vi "CRYGet Two Units Rows.vi"(6 "Phase":bool[](array[boolean]), 8 "pGraph VI In":refnum<vi>, 9 "New Rows In":i32[](array[numeric]), 10 "Old Rows In":i32[](array[numeric]), 11 "Type":enum16{"Curves", "Values", "Results", "WFM"}(ring)) -> (0 "Unit2":string, 1 "Unit1":string, 3 "All Rows Out":i32[](array[numeric]), 4 "Two Units":i32, 5 "New Rows Out":i32[](array[numeric]), 7 "New Exist?":bool)   [LabVIEW 2013]
panel:
  out "Find1":bool
  out "Message":bool
  out "Find2":bool
  out "Unit Flag":i32[](array[numeric])
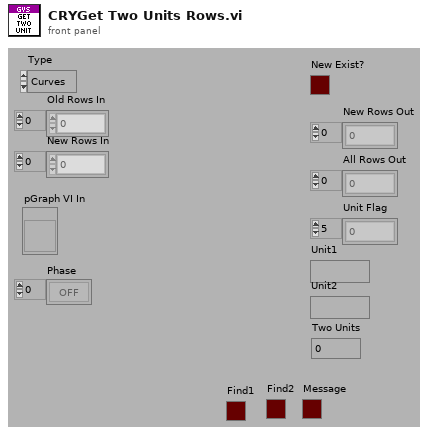
[diagram p1: front panel]
types:
  T1 = enum16{"OK", "Yes", "YesNo", "YesNoCancel", "ReplaceAppend"}
  T2 = typedef "CRYData Cluster.ctl" = cluster{"Name":string, "Curve":cluster{"x":dbl, "y":dbl, "z":dbl}[], "X data":u16, "Y data":u16, "Z data":u16, "X axis":u16, "Y axis":u16, "Z axis":u16, "X unit":string, "Y unit":string, "Z unit":string, "X dB ref":dbl, "Y dB ref":dbl, "Z dB ref":dbl, "single val":bool, "protected":bool, "display X":bool, "display Y":bool, "display Z":bool, "Test Info":string, "Step No.":i32, "Plot Settings":cluster{"Color":u32, "Interpolation":u8, "Point Style":u8, "Line Style":u8, "Point Color":u32, "Line Width":u8, "Bar Plot Style":u8, "Fill To":i16}, "AutoProtect":bool}
  T3 = typedef "CRYWaveform Cluster.ctl" = cluster{"Waveform":cluster{"X0":dbl, "dX":dbl, "Y":sgl[]}, "X data":u16, "Y data":u16, "Y axis":u16, "X unit":string, "Y unit":string, "Y dB ref":dbl, "display Y":bool, "display X":bool, "Overload?":bool, "Test Info":string, "Step No.":i32, "Name":string, "protected":bool, "Sqc history":string[], "Signal Channel ID":i32, "Plot Settings":cluster{"Color":u32, "Interpolation":u8, "Point Style":u8, "Line Style":u8, "Point Color":u32, "Line Width":u8, "Bar Plot Style":u8, "Fill To":i16}, "AutoProtect":bool}
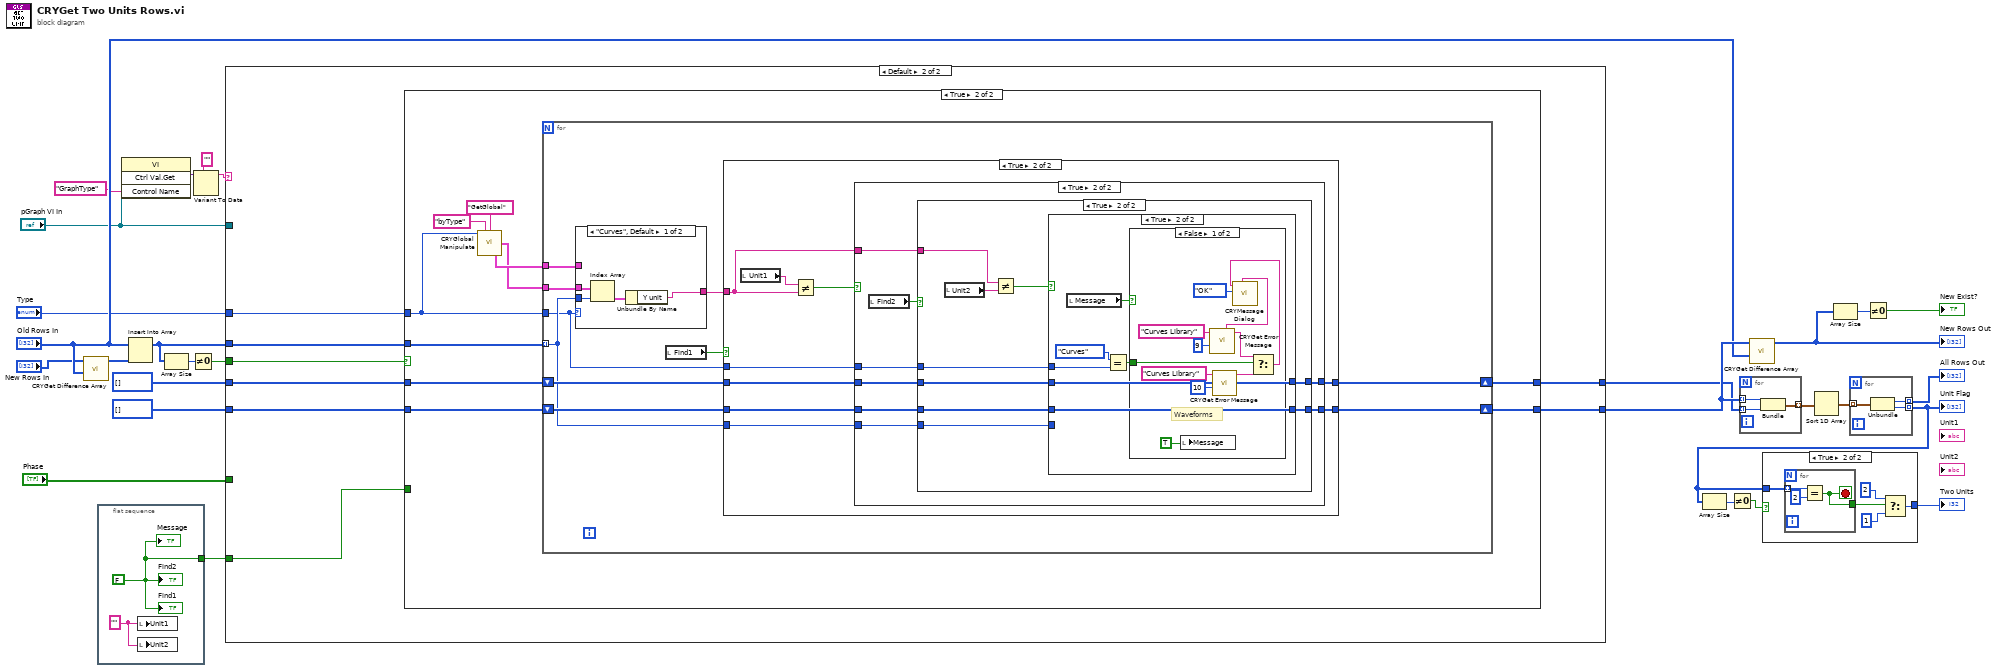
[diagram p0: block diagram]
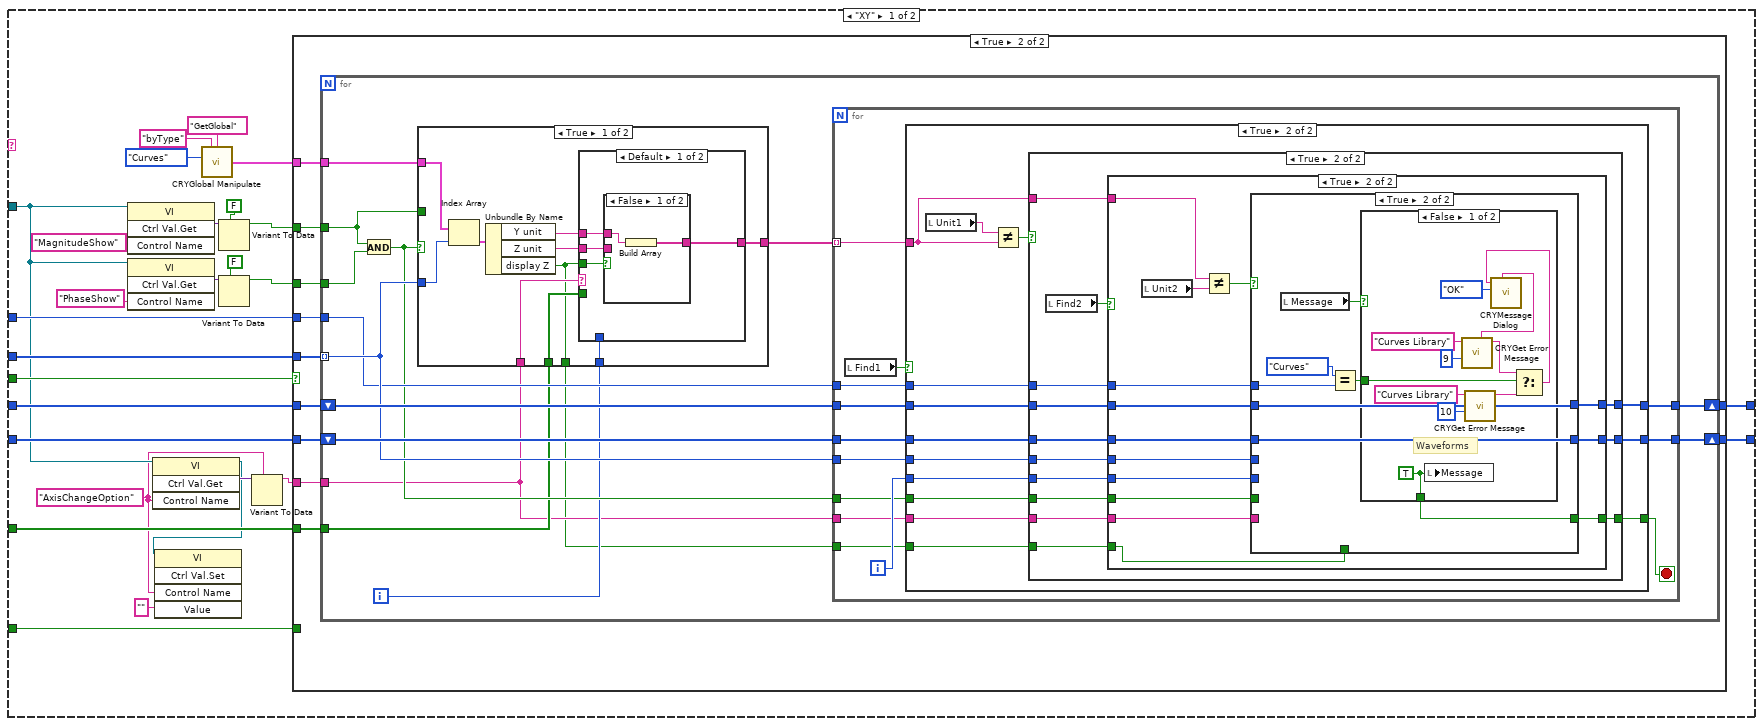
[diagram p2: hidden frame]
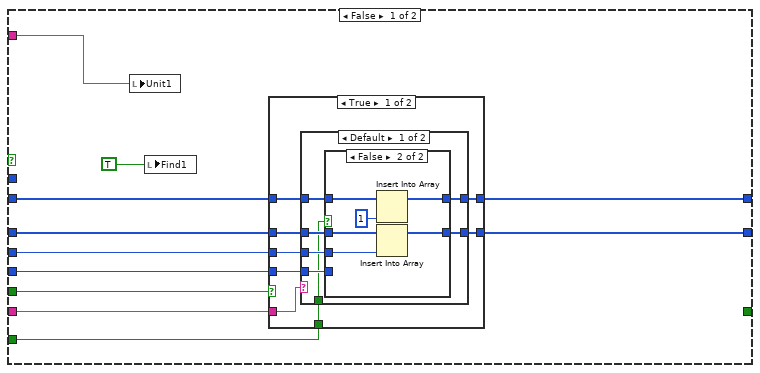
[diagram p4: hidden frame]
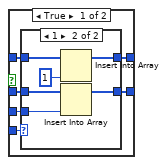
[diagram p5: hidden frame]
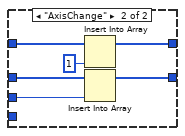
[diagram p7: hidden frame]
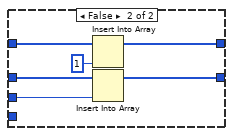
[diagram p8: hidden frame]
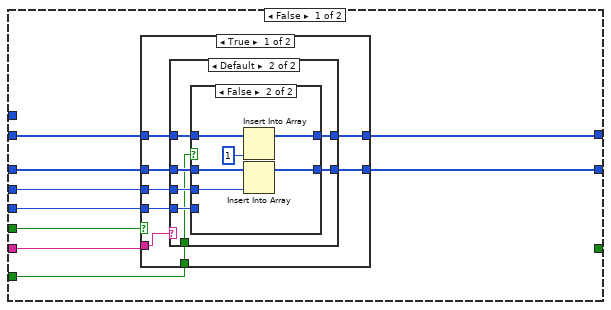
[diagram p9: hidden frame]
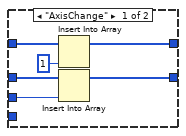
[diagram p10: hidden frame]
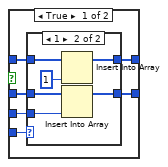
[diagram p11: hidden frame]
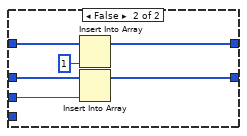
[diagram p13: hidden frame]
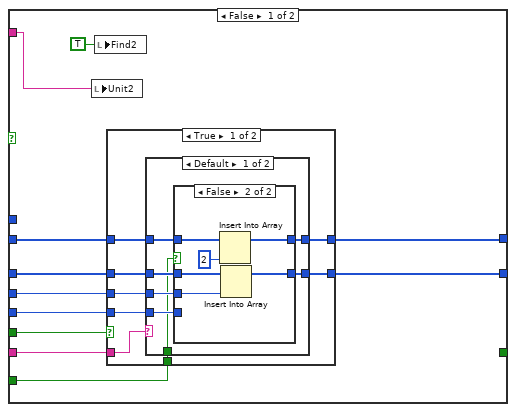
[diagram p14: hidden frame]
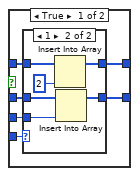
[diagram p15: hidden frame]
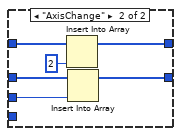
[diagram p17: hidden frame]
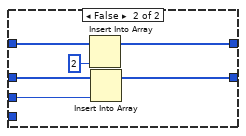
[diagram p18: hidden frame]
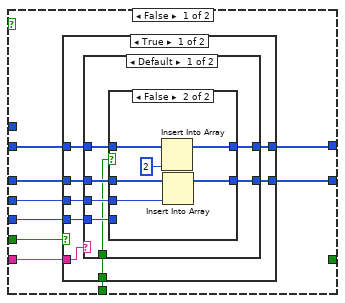
[diagram p19: hidden frame]
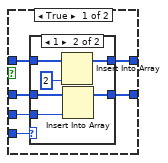
[diagram p20: hidden frame]
diagram:
  n1 = call "CRYGet Difference Array.vi"("Array 2"="Old Rows In", "Array 1"="New Rows In") -> ("Diff Out"=w16:i32[])  [unwired: 3 in, 6 out]
  n2 = flat-sequence {
    tunnel: [w30] -> w28
    frame #0 {
      w29 = "" ("Unit Y1")
      w30 = FALSE ("Find")
      n3 = local write "Unit1"(w29) -> ()
      n4 = local write "Unit2"(w29) -> ()
      "Find2" <- w30
      "Message" <- w30
      "Find1" <- w30
    }
  }
  n5 = invoke class="VI" method="Ctrl Val.Get"(reference="pGraph VI In", "Control Name"="GraphType") -> ("Get Control Value Variant"=w6:variant)  [unwired: 2 in, 3 out]
  n6 = Insert Into Array(array="Old Rows In", new element=w16) -> (w9:i32[])  [unwired: 1 in]
  n7 = Array Size(array=w9) -> (size(s)=w10:i32)
  n8 = Not Equal To 0?(x=w10) -> (x != 0?=w8:bool)
  n9 = Variant To Data(type="" ("Control Name"), Variant=w6) -> (data=w3:string)  [unwired: 1 in, 1 out]
  n10 = case shown="Default" w3 {
    tunnel: w28 -> [w57 w432]
    tunnel: i32[] [] ("Selected Row In") -> [w56 w431]
    tunnel: i32[] [] ("Selected Row In") -> [w55 w430]
    tunnel: [w54 w429] -> w23
    tunnel: [w53 w428] -> w22
    tunnel: w9 -> [w52 w427]
    tunnel: w8 -> [w51 w426]
    tunnel: "Type" -> [w50 w425]
    tunnel: "pGraph VI In" -> [w40 _]
    tunnel: "Phase" -> [w38 _]
    frame "XY" {
      w35 = "AxisChangeOption" ("Control Name")
      n11 = invoke class="VI" method="Ctrl Val.Get"(reference=w40, "Control Name"="MagnitudeShow") -> ("Get Control Value Variant"=w45:variant)  [unwired: 2 in, 3 out]
      n12 = invoke class="VI" method="Ctrl Val.Get"(reference=w40, "Control Name"="PhaseShow") -> ("Get Control Value Variant"=w46:variant)  [unwired: 2 in, 3 out]
      n13 = invoke class="VI" method="Ctrl Val.Get"(reference=w40, "Control Name"=w35) -> (reference out=w37:refnum<vi>, "Get Control Value Variant"=w41:variant)  [unwired: 2 in, 2 out]
      n14 = invoke class="VI" method="Ctrl Val.Set"(reference=w37, "Control Name"=w35, "Value"="" ("Control Name")) -> ()  [unwired: 2 in, 5 out]
      n15 = call "CRYGlobal Manipulate.vi"("Type"=enum16{"Curves", "Values", "Results", "WFM"}."Curves", "sOption"="byType", "sAction"="GetGlobal") -> ("Curves Out"=w31:T2[])  [unwired: 6 in, 6 out]
      n16 = Variant To Data(type=FALSE ("Find"), Variant=w45) -> (data=w43:bool)  [unwired: 1 in, 1 out]
      n17 = Variant To Data(type=FALSE ("Find"), Variant=w46) -> (data=w42:bool)  [unwired: 1 in, 1 out]
      n18 = Variant To Data(type=w35, Variant=w41) -> (data=w39:string)  [unwired: 1 in, 1 out]
      n19 = case shown="True" w51 {
        tunnel: w57 -> [_ _]
        tunnel: w56 -> [w58 w70]
        tunnel: w55 -> [w59 w69]
        tunnel: [w59 w68] -> w54
        tunnel: [w58 w67] -> w53
        tunnel: w52 -> [_ w66]
        tunnel: w50 -> [_ w65]
        tunnel: w43 -> [_ w63]
        tunnel: w42 -> [_ w62]
        tunnel: w31 -> [_ w64]
        tunnel: w39 -> [_ w61]
        tunnel: w38 -> [_ w60]
        frame False {
        }
        frame True {
          n20 = for {
            tunnel: w66 -> [w81] mode=indexing
            shift-right: [w84] -> w67
            shift-left: w70 -> [w85]
            shift-right: [w82] -> w68
            shift-left: w69 -> [w83]
            tunnel: w65 -> [w80]
            tunnel: w64 -> [w75]
            tunnel: w63 -> [w79]
            tunnel: w62 -> [w78]
            tunnel: w61 -> [w73]
            tunnel: w60 -> [w76]
            i -> [w74]
            n21 = And(x=w79, y=w78) -> (x .and. y?=w77:bool)
            n22 = case shown="True" w77 {
              tunnel: w81 -> [w396 w424]
              tunnel: [w395 w418] -> w72
              tunnel: w79 -> [_ w419]
              tunnel: w73 -> [w391 _]
              tunnel: w76 -> [w390 _]
              tunnel: w75 -> [w389 w417]
              tunnel: w74 -> [w388 _]
              tunnel: [w387 FALSE ("display Z")] -> w71
              frame True {
                n23 = Index Array(array=w389, index=w396) -> (element=w394:T2)
                n24 = Unbundle By Name(w394) -> ("Y unit"=w393:string, "Z unit"=w392:string, "display Z"=w387:bool)
                n25 = case shown="Default" w391 {
                  tunnel: [w400 w411] -> w395
                  tunnel: w393 -> [w399 w410]
                  tunnel: w392 -> [w398 w409]
                  tunnel: w387 -> [w397 _]
                  tunnel: w390 -> [_ w408]
                  tunnel: w388 -> [_ w406]
                  frame Default {
                    n26 = case shown="False" w397 {
                      tunnel: [w401 w403] -> w400
                      tunnel: w399 -> [w402 w404]
                      tunnel: w398 -> [_ w405]
                      frame False {
                        n27 = Build Array(w402) -> (w401:string[])
                      }
                      frame True {
                        n28 = Build Array(w404, w405) -> (w403:string[])
                      }
                    }
                  }
                  frame "AxisChange" {
                    n29 = Index Array(array=w408, index=w406) -> (element=w407:bool)
                    n30 = case shown="True" w407 {
                      tunnel: [w413 w414] -> w411
                      tunnel: w410 -> [_ w415]
                      tunnel: w409 -> [w412 _]
                      frame False {
                        n31 = Build Array(w412) -> (w413:string[])
                      }
                      frame True {
                        n32 = Build Array(w415) -> (w414:string[])
                      }
                    }
                  }
                }
              }
              frame False {
                n33 = Index Array(array=w417, index=w424) -> (element=w422:T2)
                n34 = Unbundle By Name(w422) -> ("Y unit"=w421:string, "Z unit"=w420:string)
                n35 = Select(t=w421, s=w419, f=w420) -> (s? t:f=w423:string)
                n36 = Build Array(w423) -> (w418:string[])
              }
            }
            n37 = for {
              tunnel: w85 -> [w98]
              tunnel: [w97] -> w84
              tunnel: w83 -> [w96]
              tunnel: [w95] -> w82
              tunnel: w81 -> [w94]
              tunnel: w72 -> [w93] mode=indexing
              tunnel: w80 -> [w91]
              tunnel: w77 -> [w89]
              tunnel: w73 -> [w88]
              tunnel: w71 -> [w86]
              i -> [w90]
              stop <- w87 stop-if-true
              n38 = local read "Find1"() -> (w92:bool)
              n39 = case shown="True" w92 {
                tunnel: w93 -> [w104 w170]
                tunnel: [w108 w167] -> w97
                tunnel: w98 -> [w109 w168]
                tunnel: w96 -> [w107 w166]
                tunnel: [w106 w165] -> w95
                tunnel: w94 -> [w105 w164]
                tunnel: w91 -> [_ w163]
                tunnel: w90 -> [w102 w161]
                tunnel: w89 -> [w101 w160]
                tunnel: w88 -> [w100 w159]
                tunnel: [_ w158] -> w87
                tunnel: w86 -> [w99 w157]
                frame False {
                  n40 = local write "Unit1"(w104) -> ()
                  n41 = local write "Find1"(TRUE) -> ()
                  n42 = case shown="True" w101 {
                    tunnel: w109 -> [w117 w156]
                    tunnel: [w116 w155] -> w108
                    tunnel: w107 -> [w115 w154]
                    tunnel: [w114 w153] -> w106
                    tunnel: w105 -> [w113 w152]
                    tunnel: w102 -> [w112 _]
                    tunnel: w100 -> [w111 _]
                    tunnel: w99 -> [w110 _]
                    frame True {
                      n43 = case shown="Default" w111 {
                        tunnel: w117 -> [w124 w150]
                        tunnel: [w123 w149] -> w116
                        tunnel: w115 -> [w122 w148]
                        tunnel: [w121 w147] -> w114
                        tunnel: w113 -> [w120 w146]
                        tunnel: w112 -> [w119 _]
                        tunnel: w110 -> [w118 _]
                        frame Default {
                          n44 = case shown="False" w118 {
                            tunnel: w124 -> [w130 w144]
                            tunnel: [w129 w143] -> w123
                            tunnel: w122 -> [w128 w142]
                            tunnel: [w127 w141] -> w121
                            tunnel: w120 -> [w126 w140]
                            tunnel: w119 -> [w125 _]
                            frame True {
                              n45 = case shown="1" w125 {
                                tunnel: w130 -> [w132 w138]
                                tunnel: [w132 w137] -> w129
                                tunnel: w128 -> [w131 w136]
                                tunnel: [w131 w135] -> w127
                                tunnel: w126 -> [_ w134]
                                frame 0, Default {
                                }
                                frame 1 {
                                n46 = Insert Into Array(array=w138, new element=1 ("new element/subarray")) -> (w137:i32[])  [unwired: 1 in]
                                n47 = Insert Into Array(array=w136, new element=w134) -> (w135:i32[])  [unwired: 1 in]
                                }
                              }
                            }
                            frame False {
                              n48 = Insert Into Array(array=w144, new element=1 ("new element/subarray")) -> (w143:i32[])  [unwired: 1 in]
                              n49 = Insert Into Array(array=w142, new element=w140) -> (w141:i32[])  [unwired: 1 in]
                            }
                          }
                        }
                        frame "AxisChange" {
                          n50 = Insert Into Array(array=w150, new element=1 ("new element/subarray")) -> (w149:i32[])  [unwired: 1 in]
                          n51 = Insert Into Array(array=w148, new element=w146) -> (w147:i32[])  [unwired: 1 in]
                        }
                      }
                    }
                    frame False {
                      n52 = Insert Into Array(array=w156, new element=1 ("new element/subarray")) -> (w155:i32[])  [unwired: 1 in]
                      n53 = Insert Into Array(array=w154, new element=w152) -> (w153:i32[])  [unwired: 1 in]
                    }
                  }
                }
                frame True {
                  n54 = local read "Unit1"() -> (w169:string)
                  n55 = Not Equal?(x=w169, y=w170) -> (x != y?=w162:bool)
                  n56 = case shown="True" w162 {
                    tunnel: w170 -> [_ w239]
                    tunnel: w168 -> [w179 w236]
                    tunnel: [w178 w238] -> w167
                    tunnel: w166 -> [w177 w235]
                    tunnel: [w176 w234] -> w165
                    tunnel: w164 -> [w175 w233]
                    tunnel: w163 -> [_ w232]
                    tunnel: w161 -> [w174 w231]
                    tunnel: w160 -> [w173 w230]
                    tunnel: w159 -> [w172 w229]
                    tunnel: [_ w228] -> w158
                    tunnel: w157 -> [w171 w227]
                    frame False {
                      n57 = case shown="True" w173 {
                        tunnel: w179 -> [w187 w226]
                        tunnel: [w186 w225] -> w178
                        tunnel: w177 -> [w185 w224]
                        tunnel: [w184 w223] -> w176
                        tunnel: w175 -> [w183 w222]
                        tunnel: w174 -> [w182 _]
                        tunnel: w172 -> [w181 _]
                        tunnel: w171 -> [w180 _]
                        frame True {
                          n58 = case shown="Default" w181 {
                            tunnel: w187 -> [w193 w200]
                            tunnel: [w192 w199] -> w186
                            tunnel: w185 -> [w191 w198]
                            tunnel: [w190 w197] -> w184
                            tunnel: w183 -> [w189 w196]
                            tunnel: w182 -> [_ w195]
                            tunnel: w180 -> [_ w194]
                            frame "AxisChange" {
                              n59 = Insert Into Array(array=w193, new element=1 ("new element/subarray")) -> (w192:i32[])  [unwired: 1 in]
                              n60 = Insert Into Array(array=w191, new element=w189) -> (w190:i32[])  [unwired: 1 in]
                            }
                            frame Default {
                              n61 = case shown="False" w194 {
                                tunnel: w200 -> [w206 w220]
                                tunnel: [w205 w219] -> w199
                                tunnel: w198 -> [w204 w218]
                                tunnel: [w203 w217] -> w197
                                tunnel: w196 -> [w202 w216]
                                tunnel: w195 -> [w201 _]
                                frame True {
                                n62 = case shown="1" w201 {
                                tunnel: w206 -> [w208 w213]
                                tunnel: [w208 w212] -> w205
                                tunnel: w204 -> [w207 w211]
                                tunnel: [w207 w210] -> w203
                                tunnel: w202 -> [_ w209]
                                frame 0, Default {
                                }
                                frame 1 {
                                n63 = Insert Into Array(array=w213, new element=1 ("new element/subarray")) -> (w212:i32[])  [unwired: 1 in]
                                n64 = Insert Into Array(array=w211, new element=w209) -> (w210:i32[])  [unwired: 1 in]
                                }
                                }
                                }
                                frame False {
                                n65 = Insert Into Array(array=w220, new element=1 ("new element/subarray")) -> (w219:i32[])  [unwired: 1 in]
                                n66 = Insert Into Array(array=w218, new element=w216) -> (w217:i32[])  [unwired: 1 in]
                                }
                              }
                            }
                          }
                        }
                        frame False {
                          n67 = Insert Into Array(array=w226, new element=1 ("new element/subarray")) -> (w225:i32[])  [unwired: 1 in]
                          n68 = Insert Into Array(array=w224, new element=w222) -> (w223:i32[])  [unwired: 1 in]
                        }
                      }
                    }
                    frame True {
                      n69 = local read "Find2"() -> (w237:bool)
                      n70 = case shown="True" w237 {
                        tunnel: w239 -> [w250 w310]
                        tunnel: [w247 w309] -> w238
                        tunnel: w236 -> [w248 w308]
                        tunnel: w235 -> [w246 w307]
                        tunnel: [w245 w306] -> w234
                        tunnel: w233 -> [w244 w305]
                        tunnel: w232 -> [_ w304]
                        tunnel: w231 -> [w243 w302]
                        tunnel: w230 -> [w242 w301]
                        tunnel: w229 -> [w241 w300]
                        tunnel: [_ w299] -> w228
                        tunnel: w227 -> [w240 w298]
                        frame False {
                          n71 = local write "Unit2"(w250) -> ()
                          n72 = local write "Find2"(TRUE ("Find")) -> ()
                          n73 = case shown="True" w242 {
                            tunnel: w248 -> [w258 w297]
                            tunnel: [w257 w296] -> w247
                            tunnel: w246 -> [w256 w295]
                            tunnel: [w255 w294] -> w245
                            tunnel: w244 -> [w254 w293]
                            tunnel: w243 -> [w253 _]
                            tunnel: w241 -> [w252 _]
                            tunnel: w240 -> [w251 _]
                            frame True {
                              n74 = case shown="Default" w252 {
                                tunnel: w258 -> [w265 w291]
                                tunnel: [w264 w290] -> w257
                                tunnel: w256 -> [w263 w289]
                                tunnel: [w262 w288] -> w255
                                tunnel: w254 -> [w261 w287]
                                tunnel: w253 -> [w260 _]
                                tunnel: w251 -> [w259 _]
                                frame Default {
                                n75 = case shown="False" w259 {
                                tunnel: w265 -> [w271 w285]
                                tunnel: [w270 w284] -> w264
                                tunnel: w263 -> [w269 w283]
                                tunnel: [w268 w282] -> w262
                                tunnel: w261 -> [w267 w281]
                                tunnel: w260 -> [w266 _]
                                frame True {
                                n76 = case shown="1" w266 {
                                tunnel: w271 -> [w273 w278]
                                tunnel: [w273 w277] -> w270
                                tunnel: w269 -> [w272 w276]
                                tunnel: [w272 w275] -> w268
                                tunnel: w267 -> [_ w274]
                                frame 0, Default {
                                }
                                frame 1 {
                                n77 = Insert Into Array(array=w278, new element=2 ("new element/subarray")) -> (w277:i32[])  [unwired: 1 in]
                                n78 = Insert Into Array(array=w276, new element=w274) -> (w275:i32[])  [unwired: 1 in]
                                }
                                }
                                }
                                frame False {
                                n79 = Insert Into Array(array=w285, new element=2 ("new element/subarray")) -> (w284:i32[])  [unwired: 1 in]
                                n80 = Insert Into Array(array=w283, new element=w281) -> (w282:i32[])  [unwired: 1 in]
                                }
                                }
                                }
                                frame "AxisChange" {
                                n81 = Insert Into Array(array=w291, new element=2 ("new element/subarray")) -> (w290:i32[])  [unwired: 1 in]
                                n82 = Insert Into Array(array=w289, new element=w287) -> (w288:i32[])  [unwired: 1 in]
                                }
                              }
                            }
                            frame False {
                              n83 = Insert Into Array(array=w297, new element=2 ("new element/subarray")) -> (w296:i32[])  [unwired: 1 in]
                              n84 = Insert Into Array(array=w295, new element=w293) -> (w294:i32[])  [unwired: 1 in]
                            }
                          }
                        }
                        frame True {
                          n85 = local read "Unit2"() -> (w311:string)
                          n86 = Not Equal?(x=w310, y=w311) -> (x != y?=w303:bool)
                          n87 = case shown="True" w303 {
                            tunnel: [w319 w374] -> w309
                            tunnel: w308 -> [w320 w374]
                            tunnel: [w317 w373] -> w306
                            tunnel: w307 -> [w318 w373]
                            tunnel: w305 -> [w316 _]
                            tunnel: w304 -> [_ w370]
                            tunnel: w302 -> [w315 _]
                            tunnel: w301 -> [w314 _]
                            tunnel: w300 -> [w313 _]
                            tunnel: [_ w368] -> w299
                            tunnel: w298 -> [w312 _]
                            frame False {
                              n88 = case shown="True" w314 {
                                tunnel: w320 -> [w328 w367]
                                tunnel: [w327 w366] -> w319
                                tunnel: w318 -> [w326 w365]
                                tunnel: [w325 w364] -> w317
                                tunnel: w316 -> [w324 w363]
                                tunnel: w315 -> [w323 _]
                                tunnel: w313 -> [w322 _]
                                tunnel: w312 -> [w321 _]
                                frame True {
                                n89 = case shown="Default" w322 {
                                tunnel: w328 -> [w335 w361]
                                tunnel: [w334 w360] -> w327
                                tunnel: w326 -> [w333 w359]
                                tunnel: [w332 w358] -> w325
                                tunnel: w324 -> [w331 w357]
                                tunnel: w323 -> [w330 _]
                                tunnel: w321 -> [w329 _]
                                frame Default {
                                n90 = case shown="False" w329 {
                                tunnel: w335 -> [w341 w355]
                                tunnel: [w340 w354] -> w334
                                tunnel: w333 -> [w339 w353]
                                tunnel: [w338 w352] -> w332
                                tunnel: w331 -> [w337 w351]
                                tunnel: w330 -> [w336 _]
                                frame True {
                                n91 = case shown="1" w336 {
                                tunnel: w341 -> [w343 w348]
                                tunnel: [w343 w347] -> w340
                                tunnel: w339 -> [w342 w346]
                                tunnel: [w342 w345] -> w338
                                tunnel: w337 -> [_ w344]
                                frame 0, Default {
                                }
                                frame 1 {
                                n92 = Insert Into Array(array=w348, new element=2 ("new element/subarray")) -> (w347:i32[])  [unwired: 1 in]
                                n93 = Insert Into Array(array=w346, new element=w344) -> (w345:i32[])  [unwired: 1 in]
                                }
                                }
                                }
                                frame False {
                                n94 = Insert Into Array(array=w355, new element=2 ("new element/subarray")) -> (w354:i32[])  [unwired: 1 in]
                                n95 = Insert Into Array(array=w353, new element=w351) -> (w352:i32[])  [unwired: 1 in]
                                }
                                }
                                }
                                frame "AxisChange" {
                                n96 = Insert Into Array(array=w361, new element=2 ("new element/subarray")) -> (w360:i32[])  [unwired: 1 in]
                                n97 = Insert Into Array(array=w359, new element=w357) -> (w358:i32[])  [unwired: 1 in]
                                }
                                }
                                }
                                frame False {
                                n98 = Insert Into Array(array=w367, new element=2 ("new element/subarray")) -> (w366:i32[])  [unwired: 1 in]
                                n99 = Insert Into Array(array=w365, new element=w363) -> (w364:i32[])  [unwired: 1 in]
                                }
                              }
                            }
                            frame True {
                              n100 = local read "Message"() -> (w372:bool)
                              n101 = Equal?(x=enum16{"Curves", "Values", "Results", "WFM"}."Curves" ("Type"), y=w370) -> (x = y?=w369:bool)
                              n102 = case shown="False" w372 {
                                selector: w372 -> [_ w386]
                                tunnel: w369 -> [w385 _]
                                tunnel: [w375 w386] -> w368
                                frame False {
                                w375 = TRUE
                                # "Waveforms"
                                n103 = local write "Message"(w375) -> ()
                                n104 = call "CRYGet Error Message.vi"("Error No"=9, "Kind"="Curves Library") -> ("Message"=w382:string, "Window Title"=w377:string)  [unwired: 4 in, 4 out]
                                n105 = call "CRYGet Error Message.vi"("Error No"=10, "Kind"="Curves Library") -> ("Message"=w379:string)  [unwired: 4 in, 5 out]
                                n106 = Select(t=w382, s=w385, f=w379) -> (s? t:f=w376:string)
                                n107 = call "CRYMessage Dialog.vi"("Window Title"=w377, "YesNoCancel"=T1."OK", "Message Content"=w376) -> ()  [unwired: 7 in, 2 out]
                                }
                                frame True {
                                }
                              }
                            }
                          }
                        }
                      }
                    }
                  }
                }
              }
            }
          }
        }
      }
    }
    frame Default {
      n108 = case shown="True" w426 {
        tunnel: w432 -> [_ _]
        tunnel: w431 -> [w433 w444]
        tunnel: w430 -> [w434 w443]
        tunnel: [w434 w442] -> w429
        tunnel: [w433 w441] -> w428
        tunnel: w427 -> [_ w440]
        tunnel: w425 -> [_ w436]
        frame False {
        }
        frame True {
          n109 = call "CRYGlobal Manipulate.vi"("Type"=w436, "sOption"="byType", "sAction"="GetGlobal") -> ("Curves Out"=w437:T2[], "WFM Out"=w438:T3[])  [unwired: 6 in, 5 out]
          n110 = for {
            tunnel: w437 -> [w450]
            tunnel: w440 -> [w449] mode=indexing
            shift-right: [w453] -> w441
            shift-left: w444 -> [w454]
            shift-right: [w451] -> w442
            shift-left: w443 -> [w452]
            tunnel: w436 -> [w445]
            tunnel: w438 -> [w446]
            n111 = case shown="\"Curves\", Default" w445 {
              tunnel: w450 -> [w458 _]
              tunnel: w449 -> [w457 w462]
              tunnel: [w455 w460] -> w448
              tunnel: w446 -> [_ w459]
              frame "Curves", Default {
                n112 = Index Array(array=w458, index=w457) -> (element=w456:T2)
                n113 = Unbundle By Name(w456) -> ("Y unit"=w455:string)
              }
              frame "WFM" {
                n114 = Index Array(array=w459, index=w462) -> (element=w461:T3)
                n115 = Unbundle By Name(w461) -> ("Y unit"=w460:string)
              }
            }
            n116 = local read "Find1"() -> (w447:bool)
            n117 = case shown="True" w447 {
              tunnel: w448 -> [w464 w479]
              tunnel: [w468 w476] -> w453
              tunnel: w454 -> [w469 w477]
              tunnel: w452 -> [w467 w475]
              tunnel: [w466 w474] -> w451
              tunnel: w449 -> [w465 w473]
              tunnel: w445 -> [_ w472]
              frame False {
                n118 = local write "Unit1"(w464) -> ()
                n119 = local write "Find1"(TRUE) -> ()
                n120 = Insert Into Array(array=w469, new element=1 ("new element/subarray")) -> (w468:i32[])  [unwired: 1 in]
                n121 = Insert Into Array(array=w467, new element=w465) -> (w466:i32[])  [unwired: 1 in]
              }
              frame True {
                n122 = local read "Unit1"() -> (w478:string)
                n123 = Not Equal?(x=w478, y=w479) -> (x != y?=w471:bool)
                n124 = case shown="True" w471 {
                  tunnel: w479 -> [_ w493]
                  tunnel: w477 -> [w484 w490]
                  tunnel: [w483 w492] -> w476
                  tunnel: w475 -> [w482 w489]
                  tunnel: [w481 w488] -> w474
                  tunnel: w473 -> [w480 w487]
                  tunnel: w472 -> [_ w486]
                  frame False {
                    n125 = Insert Into Array(array=w484, new element=1 ("new element/subarray")) -> (w483:i32[])  [unwired: 1 in]
                    n126 = Insert Into Array(array=w482, new element=w480) -> (w481:i32[])  [unwired: 1 in]
                  }
                  frame True {
                    n127 = local read "Find2"() -> (w491:bool)
                    n128 = case shown="True" w491 {
                      tunnel: w493 -> [w501 w509]
                      tunnel: [w497 w508] -> w492
                      tunnel: w490 -> [w498 w507]
                      tunnel: w489 -> [w496 w506]
                      tunnel: [w495 w505] -> w488
                      tunnel: w487 -> [w494 w504]
                      tunnel: w486 -> [_ w503]
                      frame False {
                        n129 = local write "Unit2"(w501) -> ()
                        n130 = local write "Find2"(TRUE ("Find")) -> ()
                        n131 = Insert Into Array(array=w498, new element=2 ("new element/subarray")) -> (w497:i32[])  [unwired: 1 in]
                        n132 = Insert Into Array(array=w496, new element=w494) -> (w495:i32[])  [unwired: 1 in]
                      }
                      frame True {
                        n133 = local read "Unit2"() -> (w510:string)
                        n134 = Not Equal?(x=w509, y=w510) -> (x != y?=w502:bool)
                        n135 = case shown="True" w502 {
                          tunnel: [w514 w522] -> w508
                          tunnel: w507 -> [w515 w522]
                          tunnel: [w512 w521] -> w505
                          tunnel: w506 -> [w513 w521]
                          tunnel: w504 -> [w511 _]
                          tunnel: w503 -> [_ w518]
                          frame False {
                            n136 = Insert Into Array(array=w515, new element=2 ("new element/subarray")) -> (w514:i32[])  [unwired: 1 in]
                            n137 = Insert Into Array(array=w513, new element=w511) -> (w512:i32[])  [unwired: 1 in]
                          }
                          frame True {
                            n138 = local read "Message"() -> (w520:bool)
                            n139 = Equal?(x=enum16{"Curves", "Values", "Results", "WFM"}."Curves" ("Type"), y=w518) -> (x = y?=w517:bool)
                            n140 = case shown="False" w520 {
                              tunnel: w517 -> [w532 _]
                              frame False {
                                # "Waveforms"
                                n141 = local write "Message"(TRUE) -> ()
                                n142 = call "CRYGet Error Message.vi"("Error No"=9, "Kind"="Curves Library") -> ("Message"=w529:string, "Window Title"=w524:string)  [unwired: 4 in, 4 out]
                                n143 = call "CRYGet Error Message.vi"("Error No"=10, "Kind"="Curves Library") -> ("Message"=w526:string)  [unwired: 4 in, 5 out]
                                n144 = Select(t=w529, s=w532, f=w526) -> (s? t:f=w523:string)
                                n145 = call "CRYMessage Dialog.vi"("Window Title"=w524, "YesNoCancel"=T1."OK", "Message Content"=w523) -> ()  [unwired: 7 in, 2 out]
                              }
                              frame True {
                              }
                            }
                          }
                        }
                      }
                    }
                  }
                }
              }
            }
          }
        }
      }
    }
  }
  n146 = for {
    tunnel: w23 -> [w536] mode=indexing
    tunnel: w22 -> [w535] mode=indexing
    tunnel: [w534] -> w25 mode=indexing
    n147 = Bundle(w536, w535) -> (w534:cluster{i32, i32})  [unwired: 1 out]
  }
  n148 = call "CRYGet Difference Array.vi"("Array 2"="Old Rows In", "Array 1"=w23) -> ("Diff Out"=w20:i32[])  [unwired: 3 in, 6 out]
  "New Rows Out" <- w20
  n149 = Sort 1D Array(array=w25) -> (sorted array=w24:cluster{i32, i32}[])
  n150 = Array Size(array=w20) -> (size(s)=w19:i32)
  n151 = for {
    tunnel: w24 -> [w539] mode=indexing
    tunnel: [w538] -> w21 mode=indexing
    tunnel: [w537] -> w14 mode=indexing
    n152 = Unbundle(w539) -> (w538:i32, w537:i32)
  }
  "Unit Flag" <- w14
  "All Rows Out" <- w21
  n153 = Array Size(array=w14) -> (size(s)=w12:i32)
  n154 = Not Equal To 0?(x=w12) -> (x != 0?=w11:bool)
  n155 = case shown="True" w11 {
    tunnel: w14 -> [_ w545]
    tunnel: [0 ("y") w542] -> w13
    frame False {
    }
    frame True {
      n156 = for {
        tunnel: w545 -> [w548] mode=indexing
        tunnel: [w546] -> w543
        stop <- w546 stop-if-true
        n157 = Equal?(x=w548, y=2) -> (x = y?=w546:bool)
      }
      n158 = Select(t=2 ("y"), s=w543, f=1 ("y")) -> (s? t:f=w542:i32)
    }
  }
  "Two Units" <- w13
  n159 = Not Equal To 0?(x=w19) -> (x != 0?=→"New Exist?":bool)
